vi "Server Error Global.vi"() -> ()   [LabVIEW 2019]
panel:
  out "Server Error":errorcluster
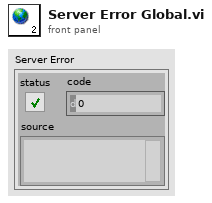
[diagram p1: front panel]
diagram:
